vi "getParameters.vi"(11 "TestForceActuatorCommand in":refnum<class "TestForceActuatorCommand.lvclass">) -> (2 "Parameters":T1, 3 "TestForceActuatorCommand out":refnum<class "TestForceActuatorCommand.lvclass">)   [LabVIEW 2016, in "TestForceActuatorCommand.lvclass"]
uses:
  TestForceActuatorCommand.lvclass
  DataTypes/Topics/CommandTestForceActuator.ctl
  DataTypes/Topics/Parts/CommandId.ctl
  TestForceActuatorCommand.lvclass/TestForceActuatorCommand.ctl
  DataTypes/Topics/M1M3SupportTopics.lvlib
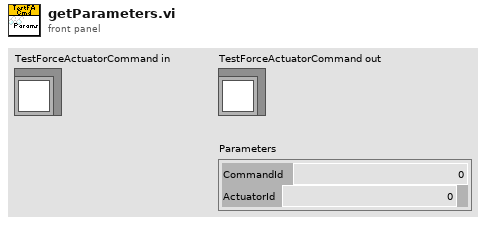
[diagram p1: front panel]
types:
  T1 = typedef "M1M3SupportTopics.lvlib/CommandTestForceActuator.ctl" = cluster{"CommandId":T2, "ActuatorId":i32}
  T2 = typedef "M1M3SupportTopics.lvlib/CommandId.ctl" = i32
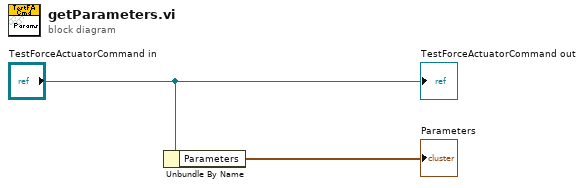
[diagram p0: block diagram]
diagram:
  n1 = Unbundle By Name("TestForceActuatorCommand in") -> ("Parameters"=→"Parameters":T1)
  "TestForceActuatorCommand out" <- "TestForceActuatorCommand in"
